vi "Read Settings.vi"(8 "error in (no error)":errorcluster, 10 "Settings ID":string, 11 "dsf refnum":T1) -> (0 "error out":errorcluster, 1 "value":T2, 3 "dsf refnum out":T1, 4 "found?":bool)   [LabVIEW 2017, in "DSF Configuration API.lvlib"]
doc: "Reads a value associated with a key in a specified section from the configuration data identified by <B>dsf refnum</B>. If the key does not exist, the VI returns the default value. This VI supports multibyte characters in strings. Wire data to the <B>default value</B> input to determine the polymorphic instance to use or manually select the instance."
uses:
  DSF Configuration API.lvlib
  Controls/DSF Settings Info.ctl
  Controls/DSF Config Data RefNum.ctl
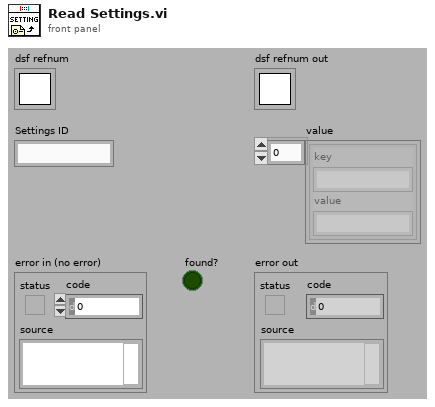
[diagram p1: front panel]
types:
  T1 = typedef "DSF Configuration API.lvlib/DSF Config Data RefNum.ctl" = refnum<k1>
  T2 = typedef "DSF Configuration API.lvlib/DSF Settings Info.ctl" = cluster{"key":string, "value":string}[]
  T3 = typedef "DSF Configuration API.lvlib/DSF Configuration Reference.ctl" = refnum<data-value>
  T4 = typedef "DSF Configuration API.lvlib/Internal.DSF Configuration.ctl" = cluster{"dsfversion":T5, "version":T5, "plugins":T6[], "groups":T9[], "transfers":T11[], "channels":T13[], "settings":T15[]}
  T5 = typedef "DSF Configuration API.lvlib/DSF Version Info.ctl" = cluster{"major":u32, "minor":u32, "fix":u32, "build":string}
  T6 = typedef "DSF Configuration API.lvlib/Internal.DSF Plugin with ID.ctl" = cluster{"id":string, "values":T7}
  T7 = typedef "DSF Configuration API.lvlib/Internal.DSF Plugin Info.ctl" = cluster{"type":string, "timing":T8, "group ids":string[], "settings id":string}
  T8 = typedef "DSF Configuration API.lvlib/DSF Timing Info.ctl" = cluster{"priority":i32, "decimation":i32, "offset":i32}
  T9 = typedef "DSF Configuration API.lvlib/Internal.DSF Group with ID.ctl" = cluster{"id":string, "values":T10}
  T10 = typedef "DSF Configuration API.lvlib/Internal.DSF Group Info.ctl" = cluster{"direction":i32, "timing":T8, "transfer ids":string[], "settings id":string}
  T11 = typedef "DSF Configuration API.lvlib/Internal.DSF Transfer with ID.ctl" = cluster{"id":string, "values":T12}
  T12 = typedef "DSF Configuration API.lvlib/Internal.DSF Transfer Info.ctl" = cluster{"byte order":i32, "channel ids":string[], "settings id":string}
  T13 = typedef "DSF Configuration API.lvlib/Internal.DSF Channel with ID.ctl" = cluster{"id":string, "values":T14}
  T14 = typedef "DSF Configuration API.lvlib/Internal.DSF Channel Info.ctl" = cluster{"count":i32, "offset":i32, "data type":i32, "resource path":string, "settings id":string}
  T15 = typedef "DSF Configuration API.lvlib/Internal.DSF Settings with ID.ctl" = cluster{"id":string, "values":T16}
  T16 = typedef "DSF Configuration API.lvlib/Internal.DSF Settings Info.ctl" = cluster{"key":string, "value":string}[]
  T17 = cluster{"dsf configuration":T4, "path":path, "dirty":bool}
  T18 = typedef "DSF Configuration API.lvlib/DSF Config Data.ctl" = cluster{"dsf configuration":T4, "path":path, "dirty":bool}
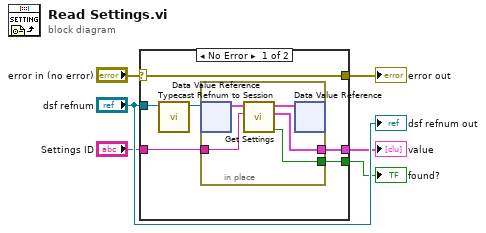
[diagram p0: block diagram]
diagram:
  n1 = case shown="No Error" "error in (no error)" {
    selector: "error in (no error)" -> [w12 w18]
    tunnel: "dsf refnum" -> [w11 _]
    tunnel: [w12 w18] -> w4
    tunnel: "Settings ID" -> [w10 _]
    tunnel: [w9 _] -> w2
    tunnel: [w8 _] -> w1
    frame No Error {
      n2 = call "Typecast Refnum to Session.vi"("dsf refnum in"=w11) -> ("DSF Configuration Session out"=w7:T3)  [unwired: 10 in]
      n3 = in-place {
        in-place-border: w10 -> [w17]
        in-place-border: [w16] -> w9
        in-place-border: [w15] -> w8
        n4 = in-place-dvr #1(w7) -> (w14:T17)  [unwired: 1 out]
        n5 = call "Get Settings.vi"("id"=w17, "DSF Configuration in"=w14) -> ("exists?"=w15:bool, "info"=w16:T2, "DSF Configuration out"=w13:T18)  [unwired: 6 in, 1 out]
        n6 = in-place-dvr #1(w13) -> ()  [unwired: 2 out]
      }
    }
    frame Error {
    }
  }
  "error out" <- w4
  "found?" <- w1
  "value" <- w2
  "dsf refnum out" <- "dsf refnum"
